vi "Restore.vi"(8 "error in (no error)":errorcluster, 9 "Previous Version":T1, 10 "Data":string, 11 "Path Selector in":refnum<class "MGI Path Selector.lvclass">) -> (0 "error out":errorcluster, 3 "Path Selector out":refnum<class "MGI Path Selector.lvclass">)   [LabVIEW 2020, in "MGI Path Selector.lvclass"]
uses:
  <userlib>/_MGI/User Interface/Path Selector XControl/Class Hierarchy/MGI Path Selector.lvclass
  <vilib>/_xctls/Version.ctl
  <userlib>/_MGI/User Interface/Path Selector XControl/Class Hierarchy/MGI Path Selector.lvclass/MGI Path Selector.ctl
  <vilib>/Utility/VariantDataType/VariantType.lvlib
  <vilib>/_xctls/XControlSupport.lvlib
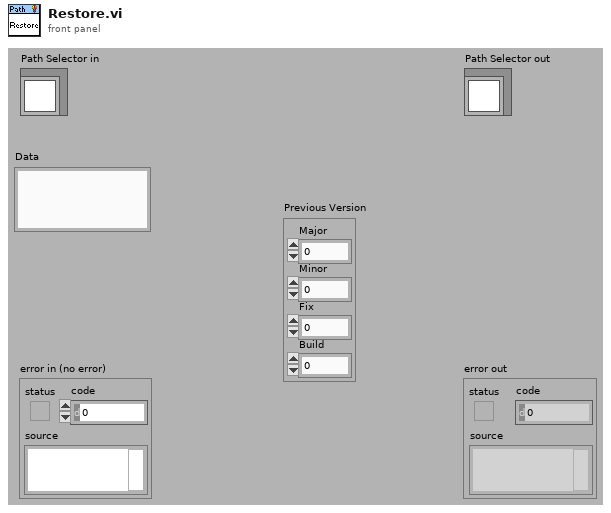
[diagram p1: front panel]
types:
  T1 = typedef "XControlSupport.lvlib/Version.ctl" = cluster{"Major":u16, "Minor":u16, "Fix":u16, "Build":u16}
  T2 = typedef "MGI Path Selector.xctl/Control Style Enum.ctl" = enum16{"System", "Modern", "Classic", "Silver"}
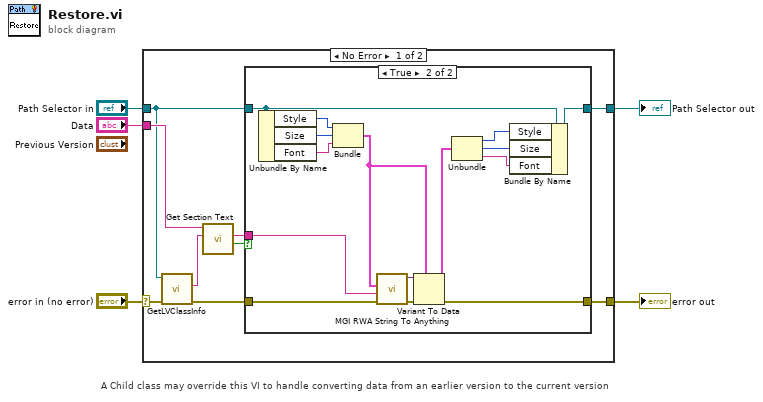
[diagram p0: block diagram]
diagram:
  # "A Child class may override this VI to handle converting data from an earlier version to the current version"
  n1 = case shown="No Error" "error in (no error)" {
    selector: "error in (no error)" -> [w14 w33]
    tunnel: [w12 w33] -> w4
    tunnel: [w7 w32] -> w2
    tunnel: "Path Selector in" -> [w6 w32]
    tunnel: "Data" -> [w11 _]
    frame No Error {
      n2 = call <vilib>:"GetLVClassInfo.vi"("error in (no error)"=w14, "Variant"=w6) -> ("error out"=w13:errorcluster, "LV Class File Name"=w10:string)  [unwired: 7 in, 1 out]
      n3 = call <userlib>:"Get Section Text.vi"("Section Name"=w10, "Data"=w11) -> ("Section Found?"=w8:bool, "Section Text"=w9:string)  [unwired: 8 in]
      n4 = case shown="True" w8 {
        tunnel: w13 -> [w15 w29]
        tunnel: [w15 w28] -> w12
        tunnel: w9 -> [_ w27]
        tunnel: w6 -> [w16 w22]
        tunnel: [w16 w21] -> w7
        frame False {
        }
        frame True {
          n5 = Unbundle By Name(w22) -> ("Style"=w24:T2, "Size"=w25:i32, "Font"=w26:string)
          n6 = Bundle("Style"=w24, "Size"=w25, "Font"=w26) -> (w23:cluster{"Style":T2, "Size":i32, "Font":string})  [unwired: 1 in]
          n7 = call <userlib>:"MGI RWA String To Anything.vi"("Error In"=w29, "String"=w27, "Type of Anything"=w23) -> ("Error Out"=w30:errorcluster, "Variant"=w31:variant)  [unwired: 6 in, 1 out]
          n8 = Variant To Data(error in=w30, type=w23, Variant=w31) -> (data=w20:cluster{"Style":T2, "Size":i32, "Font":string}, error out=w28:errorcluster)
          n9 = Unbundle(w20) -> ("Style"=w19:T2, "Size"=w18:i32, "Font"=w17:string)
          n10 = Bundle By Name(cluster=w22, "Style"=w19, "Size"=w18, "Font"=w17) -> (w21:refnum<class "MGI Path Selector.lvclass">)
        }
      }
    }
    frame Error {
    }
  }
  "error out" <- w4
  "Path Selector out" <- w2
